vi "Init.vi"(8 "error in":errorcluster, 9 "Level":T1, 10 "Name":string, 11 "Handler":refnum<class "Handler.lvclass">) -> (0 "error out":errorcluster, 3 "Handler out":refnum<class "Handler.lvclass">)   [LabVIEW 2016, in "hse-logger.lvlib" / "Handler.lvclass"]
doc: "Initiates a new Handler-object with a name and a log-level.\nThe handler processes LogRecords only if the level of the handler is greater or equal to the level of the LogRecord.\n\nReturns an errror \"500009 - Invalid parameter\" if ``Name`` is empty."
uses:
  Handler.lvclass
  LogLevel.ctl
  Handler.lvclass/Handler.ctl
  hse-logger.lvlib
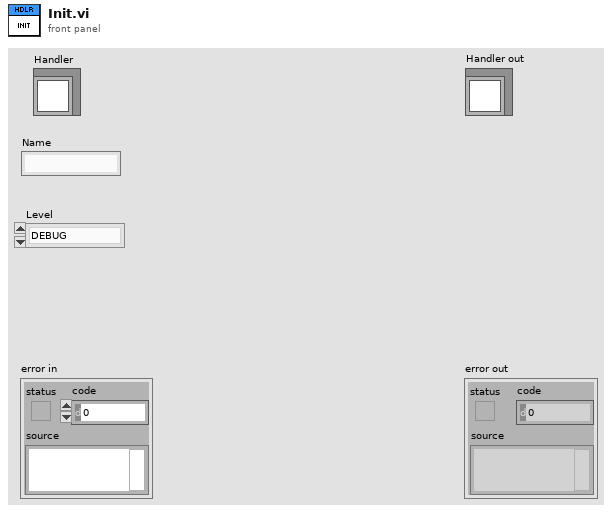
[diagram p1: front panel]
types:
  T1 = typedef "hse-logger.lvlib/LogLevel.ctl" = enum16{"DEBUG", "INFO", "WARNING", "ERROR", "CRITICAL"}
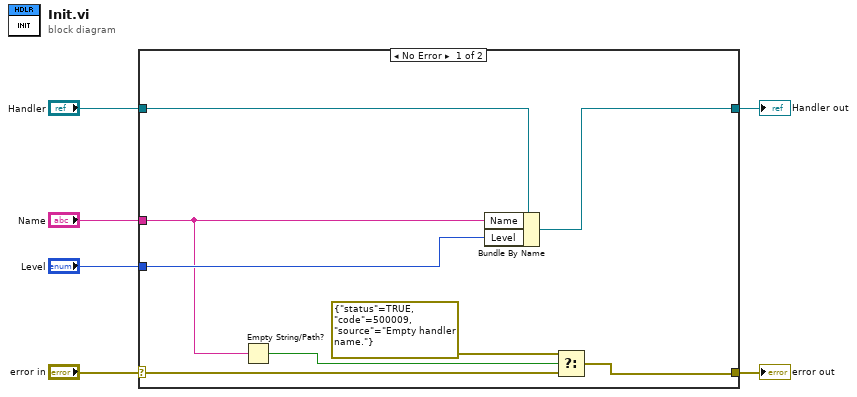
[diagram p0: block diagram]
diagram:
  n1 = case shown="No Error" "error in" {
    selector: "error in" -> [w11 w16]
    tunnel: [w10 w16] -> w5
    tunnel: [w14 w15] -> w4
    tunnel: "Name" -> [w12 _]
    tunnel: "Level" -> [w13 _]
    tunnel: "Handler" -> [w7 w15]
    frame No Error {
      n2 = Empty String/Path?(string/path=w12) -> (empty?=w9:bool)
      n3 = Bundle By Name(cluster=w7, "Name"=w12, "Level"=w13) -> (w14:refnum<class "Handler.lvclass">)
      n4 = Select(t=errorcluster {"status"=TRUE, "code"=500009, "source"="Empty handler name."}, s=w9, f=w11) -> (s? t:f=w10:errorcluster)
    }
    frame Error {
    }
  }
  "error out" <- w5
  "Handler out" <- w4
